vi "temp.vi"() -> ()   [LabVIEW 2018]
panel:
  in  "lower limit":dbl format="%#_13g"
  in  "upper limit":dbl=30.0 format="%#_13g"
  out "s? t:f":string
  out "Boolean":bool
  in  "Slide":dbl(slide) scale=0.0..100.0
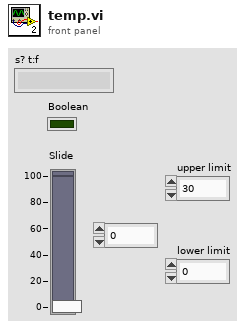
[diagram p1: front panel]
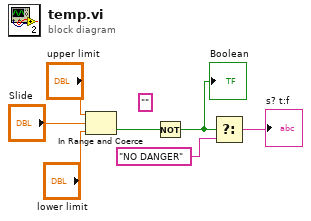
[diagram p0: block diagram]
diagram:
  (unwired) ""
  n1 = In Range and Coerce(upper limit="upper limit", x="Slide", lower limit="lower limit") -> (In Range?=w5:bool)  [unwired: 1 out]
  n2 = Not(x=w5) -> (.not. x?=w1:bool)
  "Boolean" <- w1
  n3 = Select(s=w1, f="NO DANGER") -> (s? t:f=→"s? t:f":string)  [unwired: 1 in]
